vi "1_Oscilloscope_Capture.vi"(8 "error in (no error)":errorcluster, 11 "VISA Resource Name":refnum<visa-resource-name>) -> (0 "error out":errorcluster, 2 "Waveform Graph":waveform(dbl)[](graph), 3 "VISA resource name out":refnum<visa-resource-name>)   [LabVIEW 2020]
uses:
  <instrlib>/Tektronix DPO MSO 2000 4000 Series/Public/Data/Data_Low Level/Fetch Waveform (Waveform Data Type).vi
  <instrlib>/Tektronix DPO MSO 2000 4000 Series/Tektronix DPO MSO 2000 4000 Series.lvlib
panel:
  in  "Channel 4":u16(ring)=3 items=["Channel 1", "Channel 2", "Channel 3", "Channel 4", "Math", "Reference 1", "Reference 2", "Reference 3", "Reference 4", "D0", "D1", "D2", "D3", "D4", "D5", "D6", "D7", "D8", "D9", "D10", "D11", "D12", "D13", "D14", "D15", "Amplitude", "Frequency", "Phase", "Normal", "Average", "Maximum Peak Hold", "Minimum Peak Hold"]
  in  "Channel 2":u16(ring)=1 items=["Channel 1", "Channel 2", "Channel 3", "Channel 4", "Math", "Reference 1", "Reference 2", "Reference 3", "Reference 4", "D0", "D1", "D2", "D3", "D4", "D5", "D6", "D7", "D8", "D9", "D10", "D11", "D12", "D13", "D14", "D15", "Amplitude", "Frequency", "Phase", "Normal", "Average", "Maximum Peak Hold", "Minimum Peak Hold"]
  in  "Channel 3":u16(ring)=2 items=["Channel 1", "Channel 2", "Channel 3", "Channel 4", "Math", "Reference 1", "Reference 2", "Reference 3", "Reference 4", "D0", "D1", "D2", "D3", "D4", "D5", "D6", "D7", "D8", "D9", "D10", "D11", "D12", "D13", "D14", "D15", "Amplitude", "Frequency", "Phase", "Normal", "Average", "Maximum Peak Hold", "Minimum Peak Hold"]
  in  "Channel 1":u16(ring) items=["Channel 1", "Channel 2", "Channel 3", "Channel 4", "Math", "Reference 1", "Reference 2", "Reference 3", "Reference 4", "D0", "D1", "D2", "D3", "D4", "D5", "D6", "D7", "D8", "D9", "D10", "D11", "D12", "D13", "D14", "D15", "Amplitude", "Frequency", "Phase", "Normal", "Average", "Maximum Peak Hold", "Minimum Peak Hold"]
  in  "Maximum Time (10000ms)":u32=10000
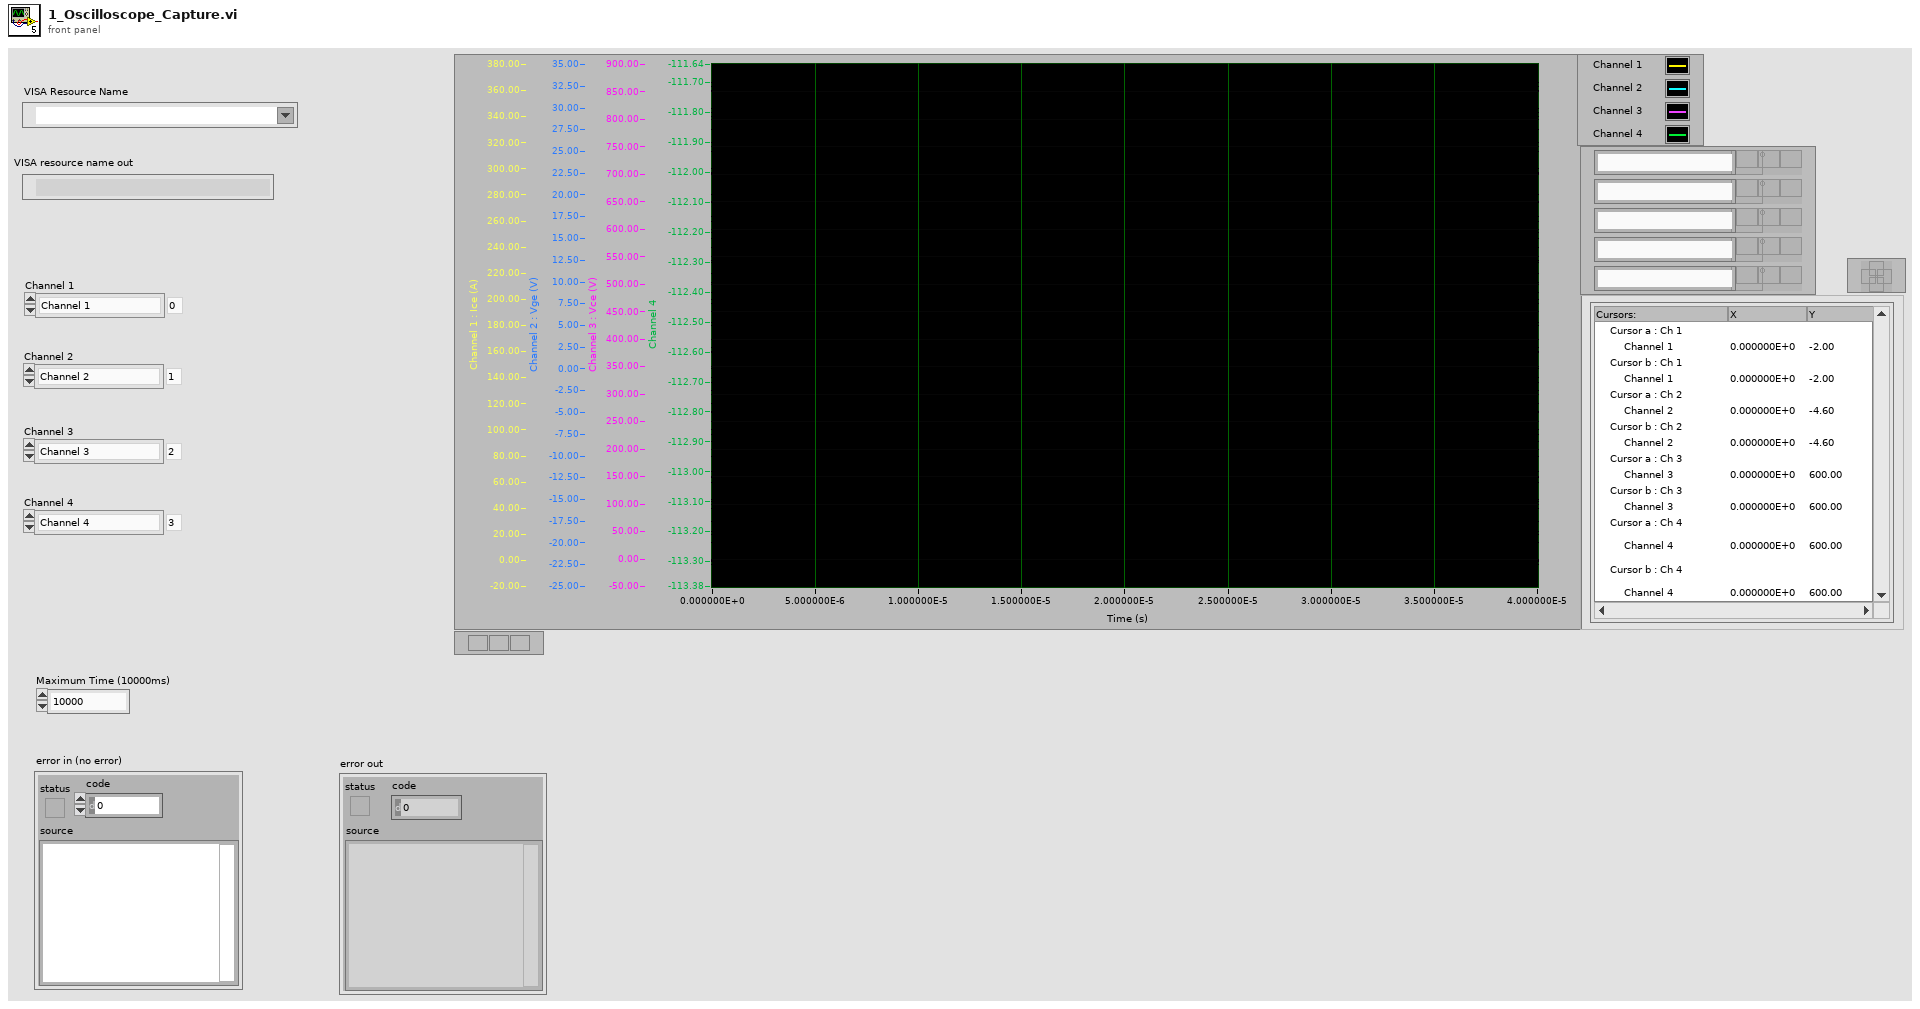
[diagram p1: front panel]
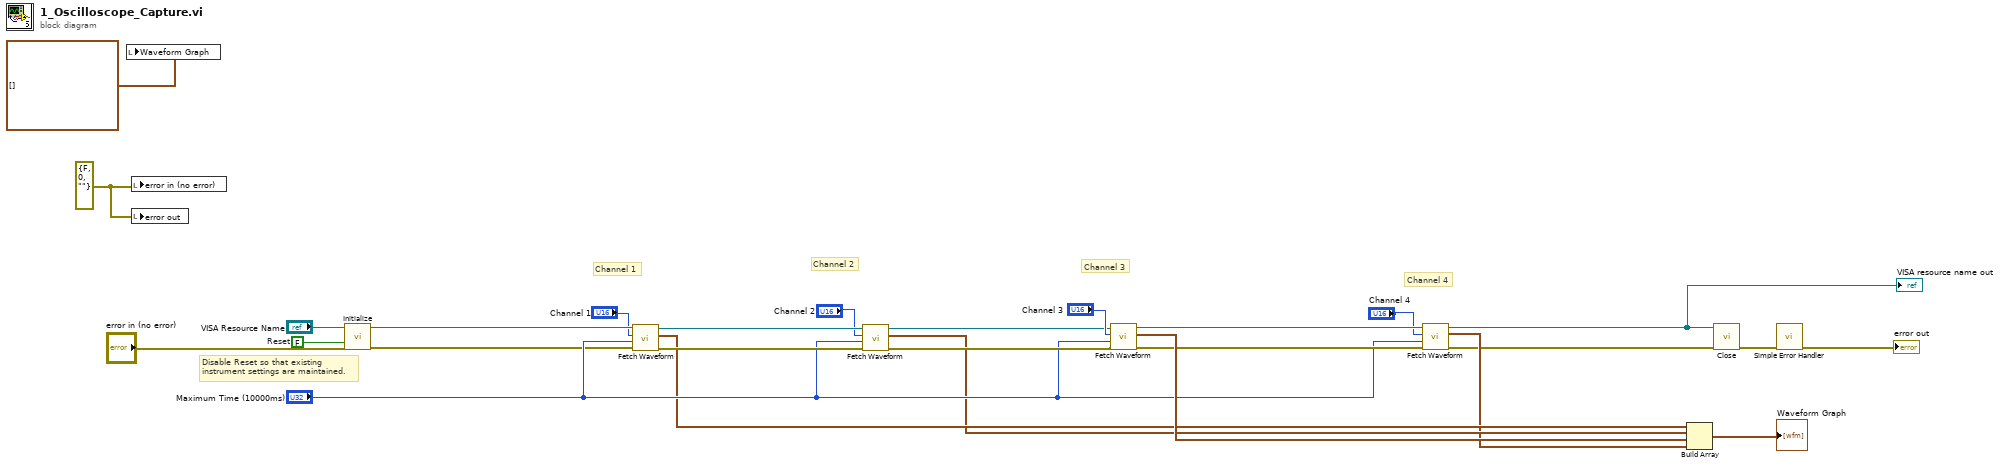
[diagram p0: block diagram]
diagram:
  w19 = errorcluster {"status"=FALSE, "code"=0, "source"=""} ("error in (no error)")
  w25 = FALSE  # Reset
  # "Channel 4"
  # "Channel 2"
  # "Channel 3"
  # "Channel 1"
  # "Disable Reset so that existing\ninstrument settings are maintained."
  n1 = local write "Waveform Graph"(waveform(dbl)[] [] ("Waveform Graph")) -> ()
  n2 = local write "error in (no error)"(w19) -> ()
  n3 = local write "error out"(w19) -> ()
  n4 = call <instrlib>:"Initialize.vi"("error in (no error)"="error in (no error)", "Reset (True)"=w25, "VISA resource name"="VISA Resource Name") -> ("error out"=w2:errorcluster, "VISA resource name out"=w24:refnum<visa-resource-name>)  [unwired: 7 in]
  n5 = call-poly <instrlib>:"Fetch Waveform.vi"("error in (no error)"=w2, "Maximum Time (10000ms)"="Maximum Time (10000ms)", "Channel (0: Channel 1)"="Channel 1", "VISA resource name"=w24) -> ("error out"=w16:errorcluster, "Waveform Data"=w6:waveform(dbl), "VISA resource name out"=w15:refnum<visa-resource-name>)  [unwired: 5 in]
  n6 = call-poly <instrlib>:"Fetch Waveform.vi"("error in (no error)"=w16, "Maximum Time (10000ms)"="Maximum Time (10000ms)", "Channel (0: Channel 1)"="Channel 2", "VISA resource name"=w15) -> ("error out"=w13:errorcluster, "Waveform Data"=w5:waveform(dbl), "VISA resource name out"=w12:refnum<visa-resource-name>)  [unwired: 5 in]
  n7 = call-poly <instrlib>:"Fetch Waveform.vi"("error in (no error)"=w13, "Maximum Time (10000ms)"="Maximum Time (10000ms)", "Channel (0: Channel 1)"="Channel 3", "VISA resource name"=w12) -> ("error out"=w11:errorcluster, "Waveform Data"=w17:waveform(dbl), "VISA resource name out"=w10:refnum<visa-resource-name>)  [unwired: 5 in]
  n8 = call-poly <instrlib>:"Fetch Waveform.vi"("error in (no error)"=w11, "Maximum Time (10000ms)"="Maximum Time (10000ms)", "Channel (0: Channel 1)"="Channel 4", "VISA resource name"=w10) -> ("error out"=w3:errorcluster, "Waveform Data"=w4:waveform(dbl), "VISA resource name out"=w8:refnum<visa-resource-name>)  [unwired: 5 in]
  "VISA resource name out" <- w8
  n9 = Build Array(w6, w5, w17, w4) -> (→"Waveform Graph":waveform(dbl)[])
  n10 = call <instrlib>:"Close.vi"("error in (no error)"=w3, "VISA resource name"=w8) -> ("error out"=w26:errorcluster)  [unwired: 9 in]
  n11 = call <vilib>:"Simple Error Handler.vi"("error in (no error)"=w26) -> ("error out"=→"error out":errorcluster)  [unwired: 4 in, 4 out]
